vi "Actuation_And_Measurement.vi"(0 "VISA resource name":refnum<visa-resource-name>, 1 "Direction":bool, 2 "Cal Param":sgl[](array[numeric]), 3 "error in (no error)":errorcluster, 4 "Motor relative position":dbl(knob) min=0.0 max=199.9 scale=0.0..199.9, 5 "Zero Offset":sgl, 6 "Samples per position":i32, 7 "Fullscale":sgl) -> (9 "End operation":bool, 11 "Position Reference":dbl, 12 "VISA resource name out":refnum<visa-resource-name>, 13 "Progress":u8(slide) scale=0.0..100.0, 14 "Monitor":T1, 15 "PLC Sensor":dbl, 16 "error out":errorcluster, 17 "Motor Ready":bool, 18 "Arduino Sensor":dbl, 19 "Communication\nAcknowledged":bool)   [LabVIEW 2018]
uses:
  <vilib>/OPCUA/controls/NodeId.ctl
  Main_SubVI/Progress.vi
  <vilib>/OPCUA/NI OPC UA Client.lvlib
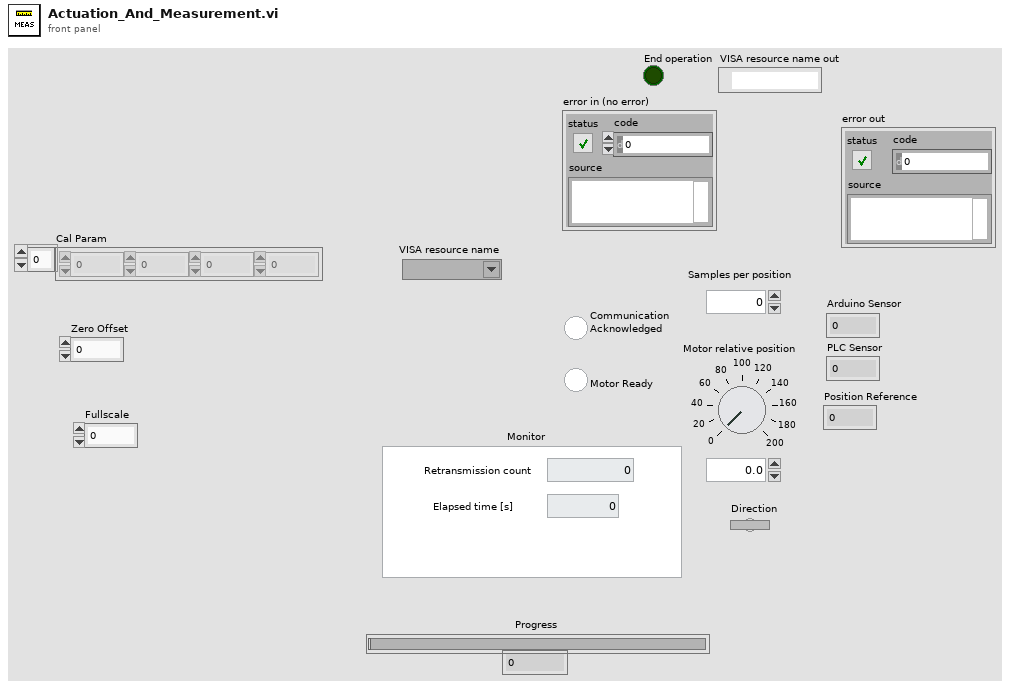
[diagram p1: front panel]
types:
  T1 = cluster{"Elapsed time [s]":dbl, "Retransmission count":dbl}
  T2 = cluster{"message mode":enum16{"None", "Sign", "Sign and Encrypt"}, "security":enum16{"Basic256", "Basic128Rsa15"}}
  T3 = typedef "NodeId.ctl" = string
  T4 = typedef "OPC UA Client Refnum.ctl" = refnum<k21>
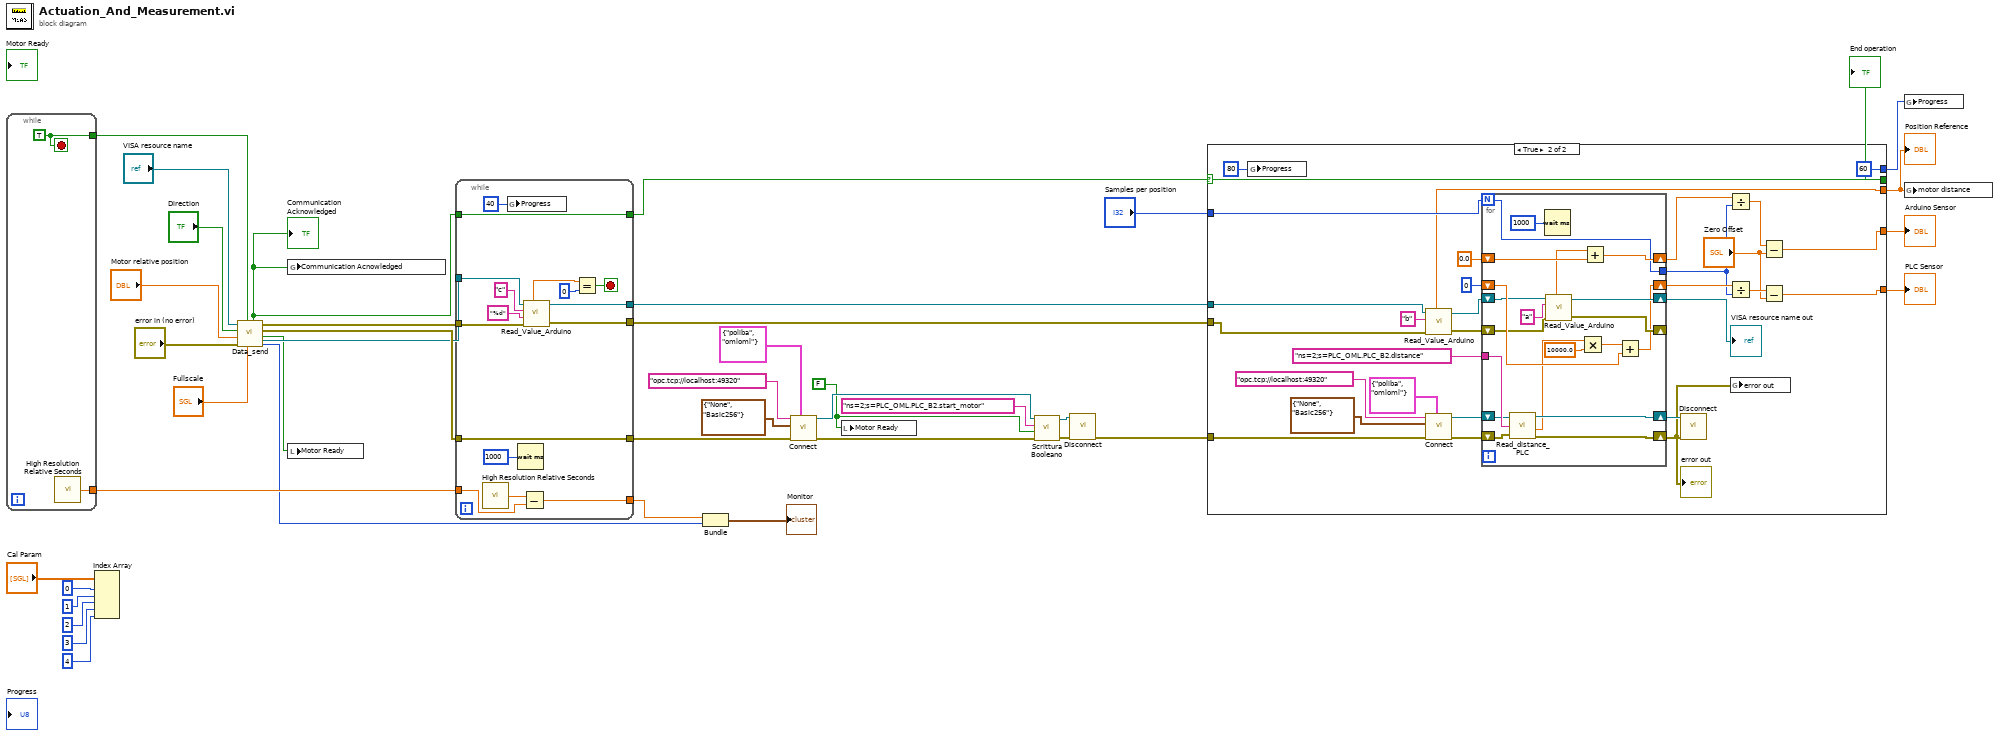
[diagram p0: block diagram]
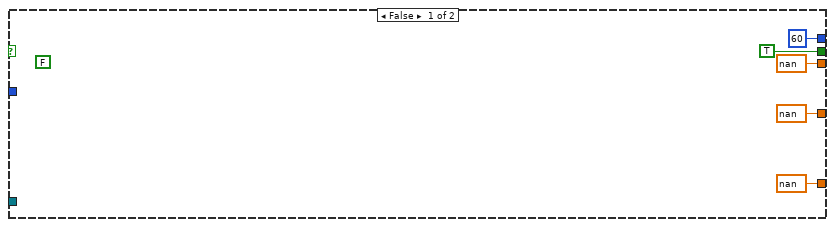
[diagram p2: hidden frame]
diagram:
  w5 = FALSE ("Value")
  n1 = while {
    tunnel: [w42] -> w41
    tunnel: [w43] -> w38
    stop <- w42 stop-if-true
    w42 = TRUE
    n2 = call <vilib>:"High Resolution Relative Seconds.vi"() -> ("relative seconds"=w43:dbl)
  }
  n3 = Index Array(array="Cal Param", index #1=0 ("index"), index #2=1 ("index"), index #3=2 ("index"), index #4=3 ("index"), index #5=4 ("index")) -> ()  [unwired: 5 out]
  n4 = call "Data_send.vi"("Full Scale"="Fullscale", "Start_communication"=w41, "error in (no error)"="error in (no error)", "Relative Motor position PLC"="Motor relative position", "Direction"="Direction", "VISA resource name"="VISA resource name") -> ("Retransmission count"=w16:i32, "Motor ready"=w6:bool, "PLC error out"=w34:errorcluster, "Arduino error out"=w32:errorcluster, "VISA resource name out"=w33:refnum<visa-resource-name>, "Communication Acnowledge"=w4:bool)
  "Communication\nAcknowledged" <- w4
  n5 = global write "Progress.vi" "Communication Acnowledged"(w4) -> ()
  n6 = local write "Motor Ready"(w6) -> ()
  n7 = while {
    tunnel: [w50] -> w17
    tunnel: w38 -> [w55]
    tunnel: w32 -> [w47]
    tunnel: [w54] -> w19
    tunnel: [w53] -> w18
    tunnel: [w52] -> w24
    tunnel: w34 -> [w52]
    tunnel: [w51] -> w7
    tunnel: w4 -> [w51]
    tunnel: w33 -> [w48]
    stop <- w57 stop-if-true
    n8 = call <vilib>:"High Resolution Relative Seconds.vi"() -> ("relative seconds"=w58:dbl)
    n9 = global write "Progress.vi" "Progress"(u8 40 ("Progress")) -> ()
    n10 = Wait (ms)(milliseconds to wait=u32 1000) -> ()  [unwired: 1 out]
    n11 = Subtract(x=w58, y=w55) -> (x-y=w50:dbl)
    n12 = call "Read_Value_Arduino.vi"("VISA resource name"=w48, "write buffer"="c", "format string (%.;%f)"="%d" ("format string"), "error in (no error)"=w47) -> ("output"=w46:dbl, "VISA resource name out"=w54:refnum<visa-resource-name>, "error out"=w53:errorcluster)  [unwired: 1 out]
    n13 = Equal?(x=w46, y=0) -> (x = y?=w57:bool)
  }
  n14 = Bundle(w17, "Retransmission count"=w16) -> (→"Monitor":cluster{dbl, "Retransmission count":i32})  [unwired: 1 in]
  n15 = call <vilib>:"Connect.vi"("username/password"=cluster{"username":string, "password":string} {"username"="poliba", "password"="omloml"}, "error in (no error)"=w24, "security policy"=T2 {"message mode"=enum."None", "security"=enum."Basic256"}, "server endpoint URL"="opc.tcp://localhost:49320") -> ("error out"=w22:errorcluster, "OPC UA client refnum out"=w23:T4)  [unwired: 5 in, 1 out]
  n16 = local write "Motor Ready"(w5) -> ()
  n17 = call "Scrittura Booleano.vi"("OPC UA client refnum in"=w23, "node ID"=T3 "ns=2;s=PLC_OML.PLC_B2.start_motor", "Value"=w5, "error in (no error)"=w22) -> ("OPC UA client refnum out"=w29:T4, "error out"=w30:errorcluster)  [unwired: 1 in, 1 out]
  n18 = call <vilib>:"Disconnect.vi"("error in (no error)"=w30, "OPC UA client refnum in"=w29) -> ("error out"=w28:errorcluster)  [unwired: 9 in]
  n19 = case shown="True" w7 {
    selector: w7 -> [_ w78]
    tunnel: [nan w72] -> w36
    tunnel: [nan w71] -> w35
    tunnel: [nan w66] -> w3
    tunnel: "Samples per position" -> [_ w79]
    tunnel: w19 -> [_ w76]
    tunnel: w18 -> [_ w75]
    tunnel: [TRUE w78] -> w1
    tunnel: w28 -> [_ w77]
    tunnel: [u8 60 ("Progress") u8 60 ("Progress")] -> w9
    frame False {
      (unwired) FALSE
    }
    frame True {
      n20 = global write "Progress.vi" "Progress"(u8 80 ("Progress")) -> ()
      n21 = call "Read_Value_Arduino.vi"("VISA resource name"=w76, "write buffer"="b", "error in (no error)"=w75) -> ("output"=w66:dbl, "VISA resource name out"=w87:refnum<visa-resource-name>, "error out"=w86:errorcluster)  [unwired: 1 in, 1 out]
      n22 = call <vilib>:"Connect.vi"("username/password"=cluster{"username":string, "password":string} {"username"="poliba", "password"="omloml"}, "error in (no error)"=w77, "security policy"=T2 {"message mode"=enum."None", "security"=enum."Basic256"}, "server endpoint URL"="opc.tcp://localhost:49320") -> ("error out"=w90:errorcluster, "OPC UA client refnum out"=w89:T4)  [unwired: 5 in, 1 out]
      n23 = for {
        N: w79 -> [w103]
        tunnel: "ns=2;s=PLC_OML.PLC_B2.distance" ("Node ID") -> [w112]
        shift-right: [w109] -> w65
        shift-left: w90 -> [w111]
        shift-right: [w108] -> _
        shift-left: w86 -> [w99]
        shift-right: [w107] -> w67
        shift-left: w87 -> [w100]
        shift-right: [w106] -> w85
        shift-left: w89 -> [w110]
        shift-right: [w105] -> w83
        shift-left: 0.0 -> [w104]
        tunnel: [w103] -> w80
        shift-right: [w102] -> w81
        shift-left: u8 0 -> [w101]
        n24 = call "Read_distance_PLC.vi"("OPC UA client refnum in"=w110, "Node ID"=w112, "error in (no error)"=w111) -> ("OPC UA client refnum out"=w106:T4, "value"=w96:sgl, "error out"=w109:errorcluster)  [unwired: 1 out]
        n25 = Wait (ms)(milliseconds to wait=u32 1000) -> ()  [unwired: 1 out]
        n26 = call "Read_Value_Arduino.vi"("VISA resource name"=w100, "write buffer"="a", "error in (no error)"=w99) -> ("output"=w95:dbl, "VISA resource name out"=w107:refnum<visa-resource-name>, "error out"=w108:errorcluster)  [unwired: 1 in, 1 out]
        n27 = Multiply(x=w96, y=10000.0) -> (x*y=w97:dbl)
        n28 = Add(x=w95, y=w104) -> (x+y=w105:dbl)
        n29 = Add(x=w97, y=w101) -> (x+y=w102:dbl)
      }
      "error out" <- w65
      "VISA resource name out" <- w67
      n30 = call <vilib>:"Disconnect.vi"("error in (no error)"=w65, "OPC UA client refnum in"=w85) -> ()  [unwired: 9 in, 1 out]
      n31 = Divide(x=w83, y=w80) -> (x/y=w69:dbl)
      n32 = Divide(x=w81, y=w80) -> (x/y=w70:dbl)
      n33 = global write "Progress.vi" "error out"(w65) -> ()
      n34 = Subtract(x=w69, y="Zero Offset") -> (x-y=w72:dbl)
      n35 = Subtract(x=w70, y="Zero Offset") -> (x-y=w71:dbl)
    }
  }
  "Arduino Sensor" <- w36
  "PLC Sensor" <- w35
  "Position Reference" <- w3
  "End operation" <- w1
  n36 = global write "Progress.vi" "Progress"(w9) -> ()
  n37 = global write "Progress.vi" "motor distance"(w3) -> ()
